vi "ListToBuffer.vi"(10 "Buffer size":u32, 11 "Input":u32[][](array[numeric])) -> (3 "Array":u32[][](array[numeric]))   [LabVIEW 2017, in "AODControl.lvlib"]
uses:
  AODControl.lvlib
panel:
  out "transposed array":u32[][](array[numeric])
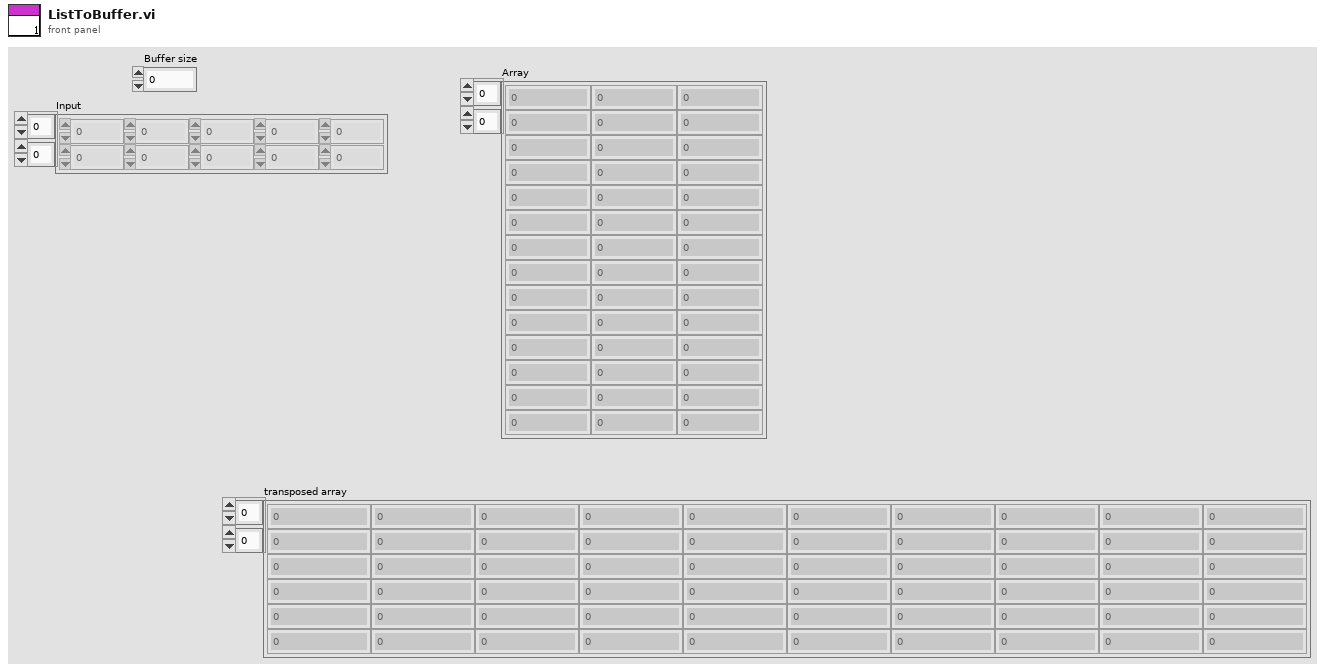
[diagram p1: front panel]
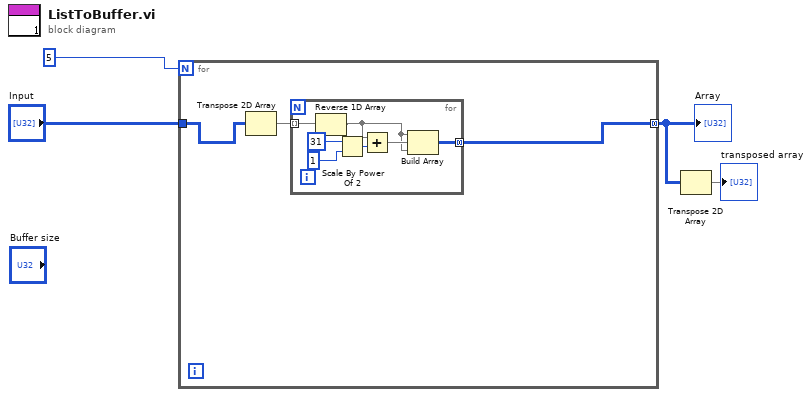
[diagram p0: block diagram]
diagram:
  n1 = for {
    N: 5 -> [_]
    tunnel: "Input" -> [w7]
    tunnel: [w6] -> w2 mode=concatenating
    n2 = Transpose 2D Array(2D array=w7) -> (transposed array=w5:u32[][])
    n3 = for {
      tunnel: w5 -> [w10] mode=indexing
      tunnel: [w11] -> w6 mode=concatenating
      n4 = Reverse 1D Array(array=w10) -> (reversed array=w8:u32[])
      n5 = Scale By Power Of 2(n=i16 31, x=u32 1 ("32bit integer")) -> (x*2^n=w14:u32)
      n6 = Add(x=w8, y=w14) -> (x+y=w9:u32[])
      n7 = Build Array(w8, w9, w8) -> (w11:u32[][])
    }
  }
  "Array" <- w2
  n8 = Transpose 2D Array(2D array=w2) -> (transposed array=→"transposed array":u32[][])
